vi "Get Config Value Path.vi"(8 "error in (no error)":errorcluster, 9 "section":string, 10 "key":string, 11 "Output Actor Hardware Interface":refnum<class "Output Actor Hardware Interface.lvclass">) -> (0 "error out":errorcluster, 1 "found?":bool, 2 "value":path, 3 "Output Actor Hardware Interface out":refnum<class "Output Actor Hardware Interface.lvclass">)   [LabVIEW 2015, in "Output Actor Hardware Interface.lvclass"]
uses:
  Output Actor Hardware Interface.lvclass
  <vilib>/Utility/config.llb/Read Key (Path).vi
  <vilib>/Utility/config.llb/NI_LVConfig.lvlib
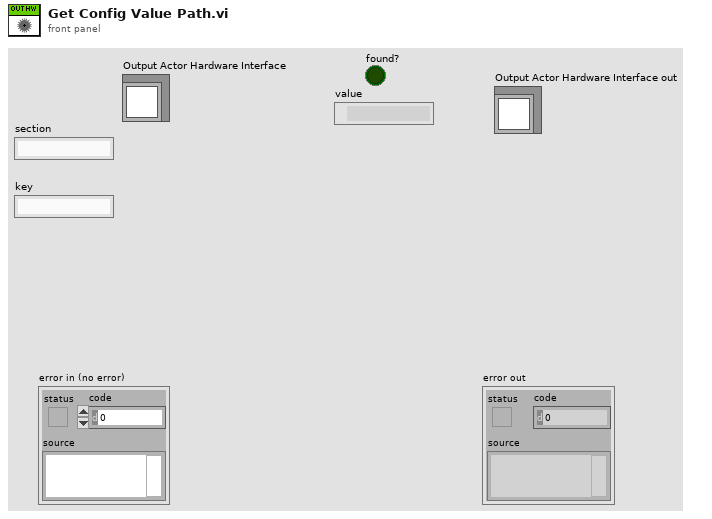
[diagram p1: front panel]
types:
  T1 = typedef "NI_LVConfig.lvlib/Config Data RefNum.ctl" = refnum<k1>
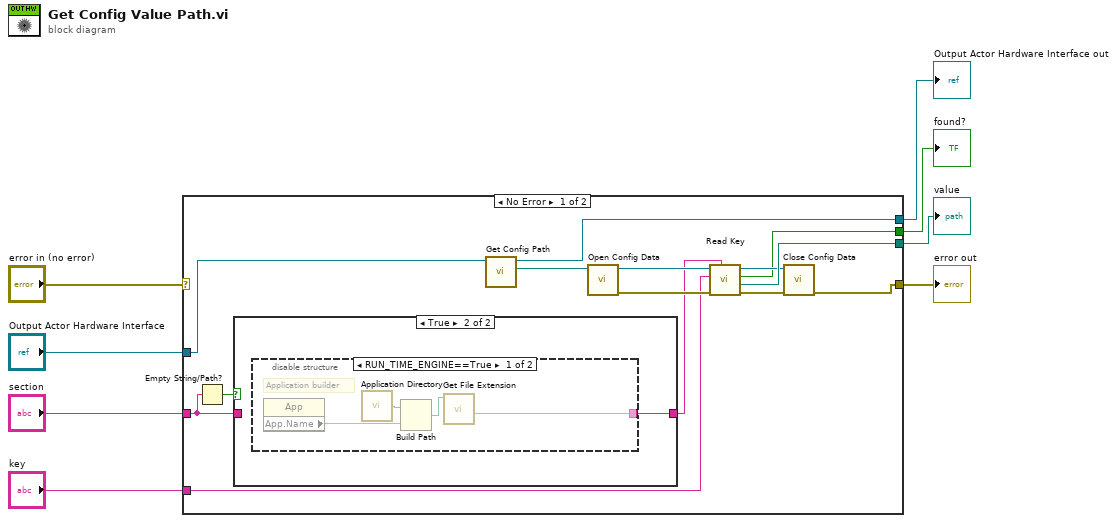
[diagram p0: block diagram]
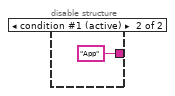
[diagram p3: hidden frame]
diagram:
  n1 = case shown="No Error" "error in (no error)" {
    selector: "error in (no error)" -> [_ w31]
    tunnel: [w10 w31] -> w7
    tunnel: [w12 w30] -> w1
    tunnel: "Output Actor Hardware Interface" -> [w14 w30]
    tunnel: [w21 _] -> w6
    tunnel: "section" -> [w15 _]
    tunnel: "key" -> [w11 _]
    tunnel: [w9 _] -> w3
    frame No Error {
      n2 = Empty String/Path?(string/path=w15) -> (empty?=w17:bool)
      n3 = case shown="True" w17 {
        tunnel: [w23 w24] -> w16
        tunnel: w15 -> [w23 _]
        frame False {
        }
        frame True {
          n4 = disable-structure shown="RUN_TIME_ENGINE==True" {
            disable-tunnel: [w25 "App" ("name or relative path")] -> w24
            frame condition #0 {
              # "Application builder"
              n5 = property class="App"() -> ("App.Name"=w28:string)  [unwired: 2 in, 2 out]
              n6 = call <vilib>:"Application Directory.vi"() -> ("Application Directory"=w27:path)
              n7 = Build Path(base path=w27, name or relative path=w28) -> (appended path=w26:path)
              n8 = call <vilib>:"Get File Extension.vi"("file"=w26) -> ("filename without extension"=w25:string)  [unwired: 6 in, 4 out]
            }
            frame condition #1 (active) {
            }
          }
        }
      }
      n9 = call "Get Config Path.vi"("Output Actor Hardware Interface.lvclass"=w14) -> ("Path"=w13:path, "Output Actor Hardware Interface.lvclass 2"=w12:refnum<class "Output Actor Hardware Interface.lvclass">)  [unwired: 9 in]
      n10 = call <vilib>:"Open Config Data.vi"("configuration file path"=w13) -> ("error out"=w19:errorcluster, "refnum"=w22:T1)  [unwired: 8 in, 1 out]
      n11 = call-poly <vilib>:"Read Key.vi"("section"=w16, "error in (no error)"=w19, "key"=w11, "refnum"=w22) -> ("error out"=w18:errorcluster, "value"=w21:path, "found?"=w9:bool, "refnum out"=w20:T1)  [unwired: 4 in]
      n12 = call <vilib>:"Close Config Data.vi"("error in (no error)"=w18, "refnum"=w20) -> ("error out"=w10:errorcluster)  [unwired: 8 in, 1 out]
    }
    frame Error {
    }
  }
  "error out" <- w7
  "found?" <- w3
  "value" <- w6
  "Output Actor Hardware Interface out" <- w1
